vi "WinCI Get Latest Version.vi"(6 "versions":string[](array[string]), 7 "advanced options":variant, 8 "error in (no error)":errorcluster, 9 "retrieval method (file)":T1 items=["file", "directory", "directory (recursive)"], 10 "files":path[](array[path]), 11 "source control reference in":T2) -> (0 "error out":errorcluster, 1 "dialog box cancelled?":bool, 2 "status message":string, 3 "source control reference out":T2)   [LabVIEW 2017, in "NI_SCC_WinCI.lvlib"]
uses:
  <vilib>/SourceControl/Providers/WinCI/NI_SCC_WinCI.lvlib
  <vilib>/SourceControl/sccapi/SCCAPI Refnum.ctl
  <vilib>/SourceControl/sccapi/SCCAPI Get Retrieval Method.ctl
  <vilib>/SourceControl/support/SCCSup Message Strings GLBL.vi
  <vilib>/SourceControl/sccapi/NI_SCC.lvlib
panel:
  out "result":i32
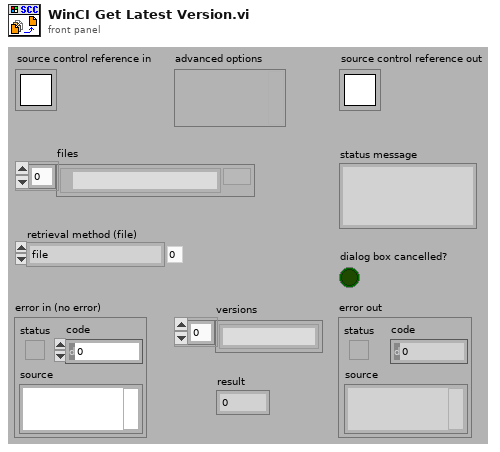
[diagram p1: front panel]
types:
  T1 = typedef "NI_SCC.lvlib/SCCAPI Get Retrieval Method.ctl" = u16
  T2 = typedef "NI_SCC.lvlib/SCCAPI Refnum.ctl" = refnum<k1>
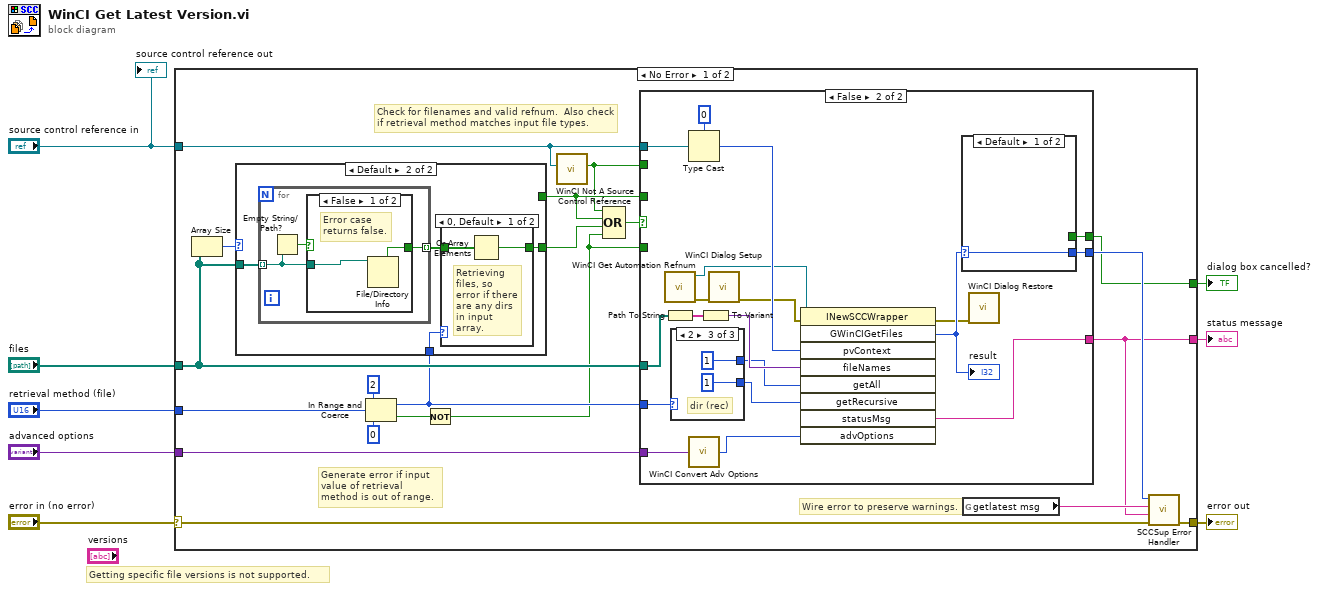
[diagram p0: block diagram]
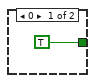
[diagram p2: hidden frame]
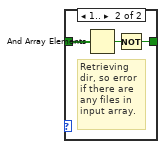
[diagram p3: hidden frame]
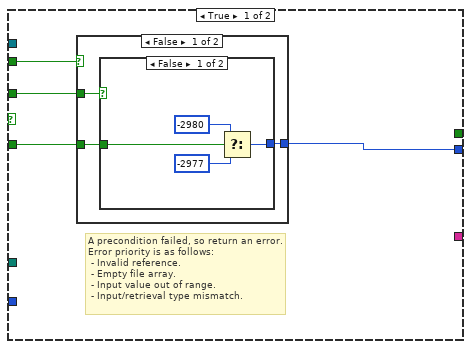
[diagram p5: hidden frame]
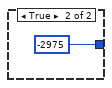
[diagram p6: hidden frame]
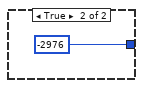
[diagram p7: hidden frame]
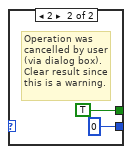
[diagram p8: hidden frame]
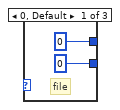
[diagram p9: hidden frame]
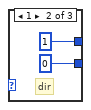
[diagram p10: hidden frame]
diagram:
  # "Getting specific file versions is not supported."
  n1 = case shown="No Error" "error in (no error)" {
    selector: "error in (no error)" -> [w16 w85]
    tunnel: [w25 w85] -> w7
    tunnel: "source control reference in" -> [w9 _]
    tunnel: [w22 _] -> w5
    tunnel: "files" -> [w20 _]
    tunnel: "retrieval method (file)" -> [w26 _]
    tunnel: [w15 _] -> w2
    tunnel: "advanced options" -> [w14 _]
    frame No Error {
      # "Generate error if input value of retrieval method is out of range."
      # "Wire error to preserve warnings."
      # "Check for filenames and valid refnum.  Also check if retrieval method matches input file types."
      n2 = Array Size(array=w20) -> (size(s)=w18:i32)
      n3 = In Range and Coerce(upper limit=u16 2, x=w26, lower limit=u16 0) -> (coerced(x)=w19:T1, In Range?=w12:bool)
      n4 = case shown="Default" w18 {
        tunnel: w20 -> [_ w33]
        tunnel: w19 -> [_ w32]
        tunnel: [_ w30] -> w17
        tunnel: [TRUE _] -> w13
        frame 0 {
        }
        frame Default {
          n5 = for {
            tunnel: w33 -> [w39] mode=indexing
            tunnel: [w41] -> w31 mode=indexing
            n6 = Empty String/Path?(string/path=w39) -> (empty?=w40:bool)
            n7 = case shown="False" w40 {
              tunnel: w39 -> [w43 _]
              tunnel: [w42 _] -> w41
              frame False {
                # "Error case returns false."
                n8 = File/Directory Info(path=w43) -> (directory=w42:bool)  [unwired: 1 in, 6 out]
              }
              frame True {
                # "Return false if empty, since node returns true on empty paths."
              }
            }
          }
          n9 = case shown="0, Default" w32 {
            tunnel: w31 -> [w35 w38]
            tunnel: [w34 w36] -> w30
            frame 0, Default {
              # "Retrieving files, so error if there are any dirs in input array."
              n10 = Or Array Elements(Boolean array=w35) -> (logical OR=w34:bool)
            }
            frame 1.. {
              # "Retrieving dir, so error if there are any files in input array."
              n11 = And Array Elements(Boolean array=w38) -> (logical AND=w37:bool)
              n12 = Not(x=w37) -> (.not. x?=w36:bool)
            }
          }
        }
      }
      n13 = Not(x=w12) -> (.not. x?=w11:bool)
      n14 = call <vilib>:"WinCI Not A Source Control Reference.vi"("source control reference in"=w9) -> ("not a source control reference?"=w10:bool)  [unwired: 1 in, 9 out]
      n15 = Compound Arithmetic op=OR(w10, w13, w17, w11) -> (w21:bool)
      n16 = case shown="False" w21 {
        tunnel: w9 -> [_ w75]
        tunnel: [_ w62] -> w22
        tunnel: w19 -> [_ w73]
        tunnel: w20 -> [_ w72]
        tunnel: [w47 w71] -> w24
        tunnel: w10 -> [w45 _]
        tunnel: w11 -> [w46 _]
        tunnel: [_ w70] -> w15
        tunnel: w14 -> [_ w69]
        tunnel: w13 -> [w44 _]
        frame True {
          # "A precondition failed, so return an error. \nError priority is as follows:\n - Invalid reference.  \n - Empty file array.\n - Input value out of range.\n - Input/retrieval type mismatch."
          n17 = case shown="False" w45 {
            tunnel: [w50 -2976 ("result")] -> w47
            tunnel: w46 -> [w49 _]
            tunnel: w44 -> [w48 _]
            frame False {
              n18 = case shown="False" w48 {
                tunnel: [w52 -2975 ("result")] -> w50
                tunnel: w49 -> [w51 _]
                frame False {
                  n19 = Select(t=-2980 ("result"), s=w51, f=-2977 ("result")) -> (s? t:f=w52:i32)
                }
                frame True {
                }
              }
            }
            frame True {
            }
          }
        }
        frame False {
          n20 = call <vilib>:"WinCI Get Automation Refnum.vi"() -> ("error out"=w58:errorcluster, "automation refnum"=w60:refnum<k7>)  [unwired: 10 out]
          n21 = Path To String(path=w72) -> (string=w68:string[])
          n22 = case shown="2" w73 {
            tunnel: [0 ("getAll") 1 ("getAll") 1 ("getAll")] -> w64
            tunnel: [0 ("getAll") 0 ("getAll") 1 ("getAll")] -> w63
            frame 0, Default {
              # "file"
            }
            frame 1 {
              # "dir"
            }
            frame 2 {
              # "dir (rec)"
            }
          }
          n23 = Type Cast(type=u32 0, x=w75) -> (*(type *) &x=w66:u32)
          n24 = call <vilib>:"WinCI Convert Adv Options.vi"("advanced options"=w69) -> ("command options"=w65:u32)  [unwired: 4 out]
          n25 = To Variant(anything=w68) -> (Variant=w67:variant)
          n26 = call <vilib>:"WinCI Dialog Setup.vi"("error in"=w58) -> ("error out"=w59:errorcluster)  [unwired: 10 out]
          n27 = invoke class="INewSCCWrapper" method="GWinCIGetFiles"(reference=w60, error in=w59, "pvContext"=w66, "fileNames"=w67, "getAll"=w64, "getRecursive"=w63, "advOptions"=w65) -> (error out=w57:errorcluster, "GWinCIGetFiles"=w61:i32, "statusMsg"=w62:string)  [unwired: 2 in, 6 out]
          "result" <- w61
          n28 = case shown="Default" w61 {
            selector: w61 -> [w76 _]
            tunnel: [w76 0 ("result")] -> w71
            tunnel: [_ TRUE] -> w70
            frame Default {
            }
            frame 2 {
              # "Operation was cancelled by user (via dialog box).  Clear result since this is a warning."
            }
          }
          n29 = call <vilib>:"WinCI Dialog Restore.vi"("error in"=w57) -> ()  [unwired: 11 out]
        }
      }
      n30 = global read "SCCSup Message Strings GLBL.vi" "getlatest msg"() -> (w23:string)
      n31 = call <vilib>:"SCCSup Error Handler.vi"("error in (no error)"=w16, "additional message"=w22, "operation message"=w23, "scc error code"=w24) -> ("error out"=w25:errorcluster)  [unwired: 7 out]
    }
    frame Error {
    }
  }
  "error out" <- w7
  "status message" <- w5
  "dialog box cancelled?" <- w2
  "source control reference out" <- "source control reference in"
